vi "Initialise.vi"(8 "error in (no error)":errorcluster, 10 "Instrument Ref":string, 11 "APS7050 in":refnum<class "APS7050.lvclass">) -> (0 "error out":errorcluster, 3 "APS7050 out":refnum<class "APS7050.lvclass">)   [LabVIEW 2021, in "Concrete.lvlib" / "APS7050.lvclass"]
uses:
  APS7050.lvclass
  APS7050.lvclass/APS7050.ctl
  Harware Abstraction/AnalogIO/Power Supply.lvclass
  <instrlib>/APS-7000 Series/APS-7000 Series.lvlib
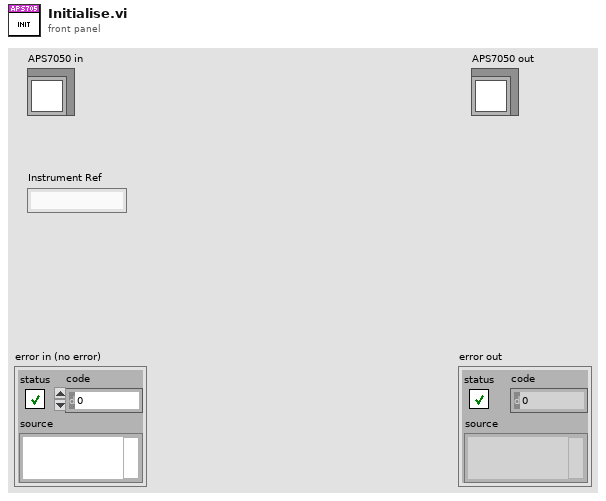
[diagram p1: front panel]
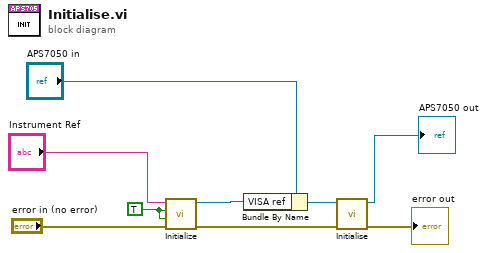
[diagram p0: block diagram]
diagram:
  w8 = TRUE ("ID Query (True)")
  n1 = call <instrlib>:"Initialize.vi"("error in (no error)"="error in (no error)", "Reset (True)"=w8, "ID Query (True)"=w8, "VISA resource name"="Instrument Ref") -> ("error out"=w6:errorcluster, "VISA resource name out"=w3:refnum<visa-resource-name>)  [unwired: 6 in]
  n2 = Bundle By Name(cluster="APS7050 in", "VISA ref"=w3) -> (w4:refnum<class "APS7050.lvclass">)
  n3 = call-parent "Initialise.vi"("error in (no error)"=w6, "Instrument in"=w4) -> ("error out"=→"error out":errorcluster, "Instrument out"=→"APS7050 out":refnum<class "APS7050.lvclass">)  [unwired: 8 in]
